vi "Pigeon Sensor Readings.vi"() -> ()   [LabVIEW 2018]
uses:
  <vilib>/Rock Robotics/WPI/ThirdParty/Phoenix-LabVIEW/Pigeon IMU/CTRE_PigeonIMU_GetYPR.vi
  <vilib>/Rock Robotics/WPI/ThirdParty/Phoenix-LabVIEW/Pigeon IMU/CTRE_PigeonIMU_GetTempStateUpTime.vi
panel:
  out "Yaw":dbl format="%#_13g"
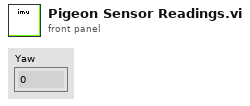
[diagram p1: front panel]
types:
  T1 = typedef "CTRE_PigeonIMU_DeviceRef.ctl" = cluster{"DeviceStatus":errorcluster, "Device Number":u8, "Type":T2, "Device ID":u32, "Handle":u64, "UsageFrame":u32, "Library Path":path}
  T2 = typedef "CTRE_PigeonIMU_ConnectionType.ctl" = u32
  T3 = typedef "CTRE_PigeonIMU_CalibrationMode.ctl" = u16
  T4 = typedef "CTRE_PigeonIMU_PigeonState.ctl" = enum16{"NoComm", "Initializing", "Ready", "UserCalibration"}
  T5 = cluster{"CurrentMode":T3, "LastCalError":i32, "CalBooting?":bool, "PigeonState":T4, "UpTime":u32, "Temp. (C)":dbl, "Temp Compensation Event Count":u32, "No Motion Event Count":u32}
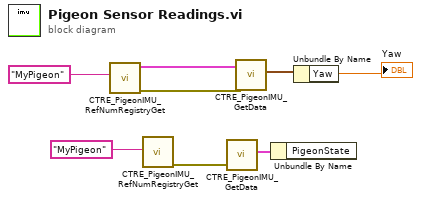
[diagram p0: block diagram]
diagram:
  n1 = call <vilib>:"CTRE_PigeonIMU_RefNumRegistryGet.vi"("refnum name"="MyPigeon") -> ("error out"=w6:errorcluster, "PigeonIMUDevRef"=w1:T1)  [unwired: 9 in]
  n2 = call <vilib>:"CTRE_PigeonIMU_RefNumRegistryGet.vi"("refnum name"="MyPigeon") -> ("error out"=w3:errorcluster)  [unwired: 9 in, 1 out]
  n3 = call-poly <vilib>:"CTRE_PigeonIMU_GetData.vi"("error in (no error)"=w3) -> ("Temp/State/UpTime"=w5:T5)  [unwired: 8 in, 2 out]
  n4 = call-poly <vilib>:"CTRE_PigeonIMU_GetData.vi"("error in (no error)"=w6, "PigeonIMUDevRef"=w1) -> ("Yaw Pitch Roll"=w8:cluster{"Yaw":dbl, "Pitch":dbl, "Roll":dbl})  [unwired: 7 in, 2 out]
  n5 = Unbundle By Name(w5) -> ()  [unwired: 1 out]
  n6 = Unbundle By Name(w8) -> ("Yaw"=→"Yaw":dbl)
